vi "Search By Name.vi"(9 "Node Name":string, 10 "Optional Unique Parent Path":string, 11 "Tree Map In":T1) -> (3 "Unique Paths Set":set{string}(c389))   [LabVIEW 2020, in "Tree Map.lvlib"]
doc: "Searches the Tree Map for nodes with a name containing the input node name string. The optional unique parent path can be specified to limit the search to one level of the tree.\n\n<b>Author:</b> Piotr Kruczkowski <PrimaryKey>\n<b>License:</b> NewBSD\n\nCopyright (c) 2019, National Instruments\nAll rights reserved.\n\nRedistribution and use in source and binary forms, with or without\nmodification, are permitted provided that the following conditions are met:\n1. Redistributions of source code must retain the above copyright\n notice, this list of conditions and the following disclaimer.\n2. Redistributions in binary form must reproduce the above copyright\n notice, this list of conditions and the following disclaimer in the\n documentation and/or other materials provided with the distribution.\n3. Neither the name of National Instruments nor the\n names of its contributors may be used to endorse or promote products\n derived from this software without specific prior written permission.\n\nTHIS SOFTWARE IS PROVIDED BY National Instruments ''AS IS'' AND ANY\nEXPRESS OR IMPLIED WARRANTIES, INCLUDING, BUT NOT LIMITED TO, THE IMPLIED\nWARRANTIES OF MERCHANTABILITY AND FITNESS FOR A PARTICULAR PURPOSE ARE\nDISCLAIMED. IN NO EVENT SHALL National Instruments BE LIABLE FOR ANY\nDIRECT, INDIRECT, INCIDENTAL, SPECIAL, EXEMPLARY, OR CONSEQUENTIAL DAMAGES\n(INCLUDING, BUT NOT LIMITED TO, PROCUREMENT OF SUBSTITUTE GOODS OR SERVICES;\nLOSS OF USE, DATA, OR PROFITS; OR BUSINESS INTERRUPTION) HOWEVER CAUSED AND\nON ANY THEORY OF LIABILITY, WHETHER IN CONTRACT, STRICT LIABILITY, OR TORT\n(INCLUDING NEGLIGENCE OR OTHERWISE) ARISING IN ANY WAY OUT OF THE USE OF THIS\nSOFTWARE, EVEN IF ADVISED OF THE POSSIBILITY OF SUCH DAMAGE."
uses:
  Tree Map.lvlib
  Tree Map Data.ctl
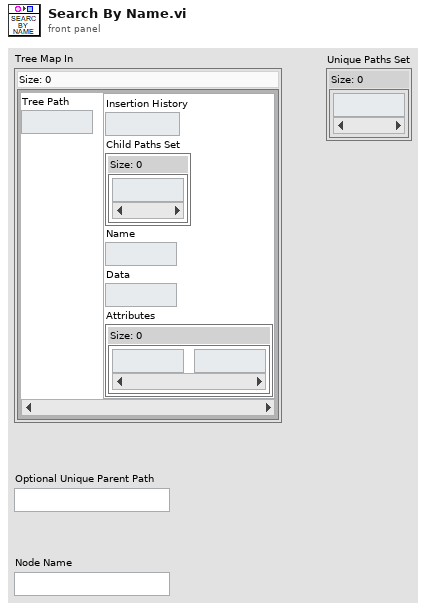
[diagram p1: front panel]
types:
  T1 = typedef "Tree Map.lvlib/Tree Map Data.ctl" = map{string, cluster{"Insertion History":i32, "Child Paths Set":set{string}, "Name":string, "Data":string, "Attributes":map{string, string}}}
  T2 = cluster{"Insertion History":i32, "Child Paths Set":set{string}, "Name":string, "Data":string, "Attributes":map{string, string}}
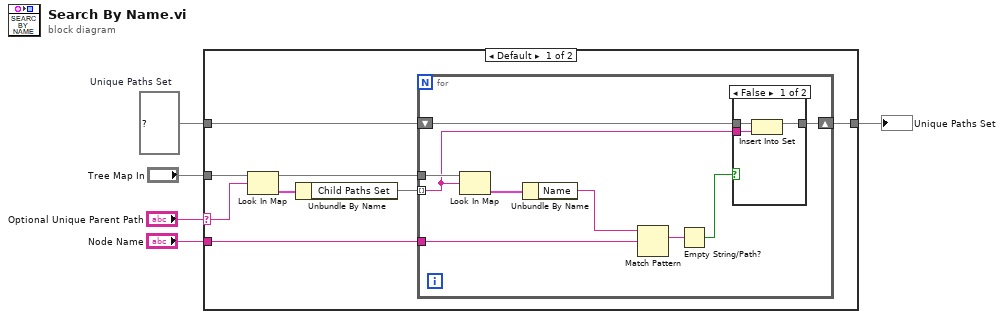
[diagram p0: block diagram]
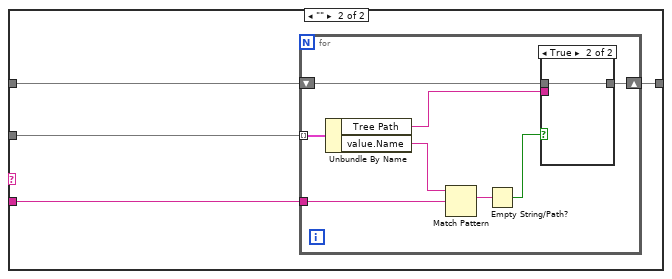
[diagram p3: hidden frame]
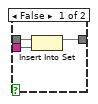
[diagram p4: hidden frame]
diagram:
  w4 = set{string} {}  # Unique Paths Set
  n1 = case shown="Default" "Optional Unique Parent Path" {
    selector: "Optional Unique Parent Path" -> [w10 _]
    tunnel: "Tree Map In" -> [w7 w29]
    tunnel: w4 -> [w12 w28]
    tunnel: [w11 w27] -> w3
    tunnel: "Node Name" -> [w6 w26]
    frame Default {
      n2 = Look In Map(map=w7, key=w10) -> (value=w9:T2)  [unwired: 1 in, 1 out]
      n3 = Unbundle By Name(w9) -> ("Child Paths Set"=w8:set{string})
      n4 = for {
        shift-right: [w21] -> w11
        shift-left: w12 -> [w20]
        tunnel: w8 -> [w13] mode=indexing
        tunnel: w7 -> [w17]
        tunnel: w6 -> [w14]
        n5 = Look In Map(map=w17, key=w13) -> (value=w16:T2)  [unwired: 1 in, 1 out]
        n6 = Unbundle By Name(w16) -> ("Name"=w15:string)
        n7 = Match Pattern(string=w15, regular expression=w14) -> (match substring=w19:string)  [unwired: 1 in, 3 out]
        n8 = Empty String/Path?(string/path=w19) -> (empty?=w18:bool)
        n9 = case shown="False" w18 {
          tunnel: w13 -> [w24 _]
          tunnel: [w23 w25] -> w21
          tunnel: w20 -> [w22 w25]
          frame False {
            n10 = Insert Into Set(10:w24, 11:w22) -> (3:w23:set{string})  [unwired: 1 out]
          }
          frame True {
          }
        }
      }
    }
    frame "" {
      n11 = for {
        tunnel: w29 -> [w37] mode=indexing
        shift-right: [w36] -> w27
        shift-left: w28 -> [w35]
        tunnel: w26 -> [w32]
        n12 = Unbundle By Name(w37) -> ("Tree Path"=w34:string, "value.Name"=w33:string)
        n13 = Match Pattern(string=w33, regular expression=w32) -> (match substring=w31:string)  [unwired: 1 in, 3 out]
        n14 = Empty String/Path?(string/path=w31) -> (empty?=w30:bool)
        n15 = case shown="True" w30 {
          tunnel: w34 -> [w40 _]
          tunnel: [w39 w41] -> w36
          tunnel: w35 -> [w38 w41]
          frame False {
            n16 = Insert Into Set(10:w40, 11:w38) -> (3:w39:set{string})  [unwired: 1 out]
          }
          frame True {
          }
        }
      }
    }
  }
  "Unique Paths Set" <- w3
